vi "ReadSoundCard.vi"(3 "All Info":T1 {"Data Set"."Settings"."Time" format="%<%H:%M\n%d/%m/%y>T"; "task ID" format="%.0x"}) -> (0 "Data Set":T2[](array[typedef]) {"Settings"."Time" format="%<%H:%M\n%d/%m/%y>T"}, 1 "All Info":T1 {"Data Set"."Settings"."Time" format="%<%H:%M\n%d/%m/%y>T"; "task ID" format="%.0x"})   [LabVIEW 2014]
uses:
  <userlib>/CurtinCode/DataControl.ctl
  <userlib>/CurtinCode/SettingsControl.ctl
  <userlib>/CurtinCode/AllDataCtrl.ctl
  <vilib>/sound2/lvsound2.llb/Sound Input Task ID.ctl
  <vilib>/DAQmx/read.llb/DAQmx Read (Analog 1D Wfm NChan NSamp).vi
  <vilib>/sound2/lvsound2.llb/Sound Input Read (DBL).vi
panel:
  out "Waveform Graph":dbl[](graph)
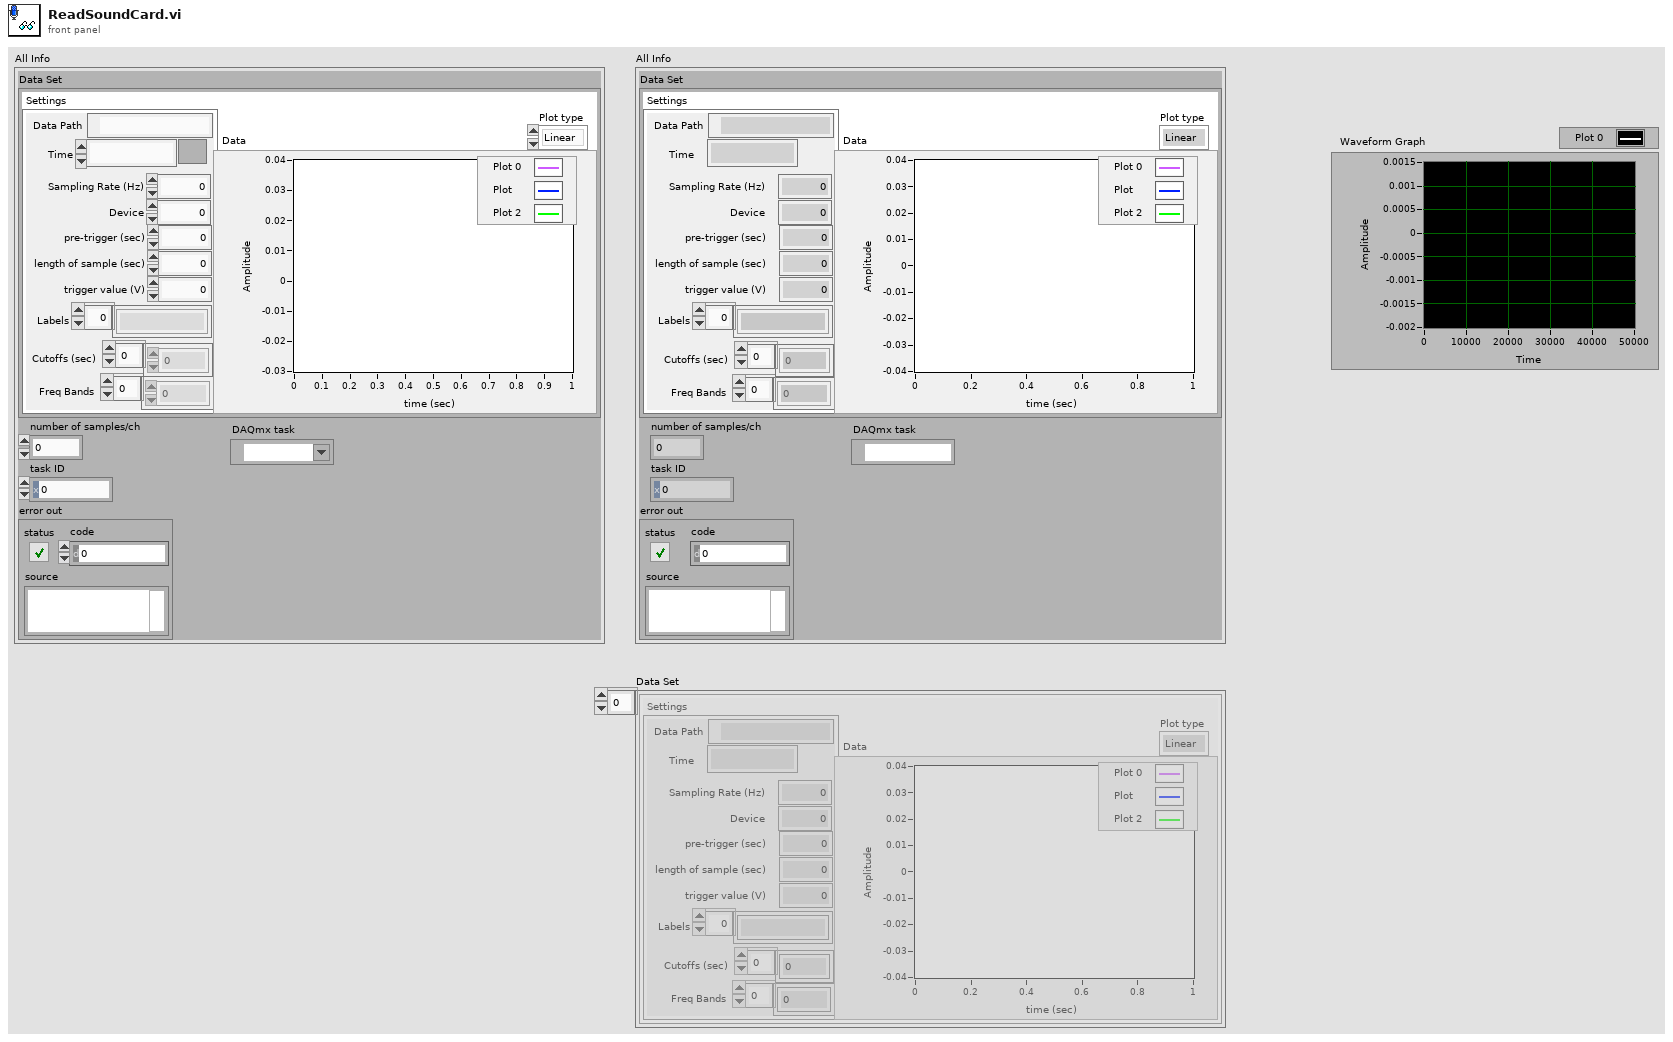
[diagram p1: front panel]
types:
  T1 = typedef "AllDataCtrl.ctl" = cluster{"Data Set":T2, "number of samples/ch":i32, "task ID":T4, "error out":errorcluster, "DAQmx task":refnum<k21>}
  T2 = typedef "DataControl.ctl" = cluster{"Settings":T3, "Data":cluster{i32, dbl, "data":dbl[]}[], "Plot type":enum16{"Linear", "log"}}
  T3 = typedef "SettingsControl.ctl" = cluster{"Data Path":path, "Time":timestamp, "Sampling Rate (Hz)":u16, "Device":u16, "pre-trigger (sec)":dbl, "length of sample (sec)":dbl, "trigger value (V)":dbl, "Labels":string[], "Cutoffs (sec)":dbl[], "Freq Bands":dbl[]}
  T4 = typedef "Sound Input Task ID.ctl" = u32
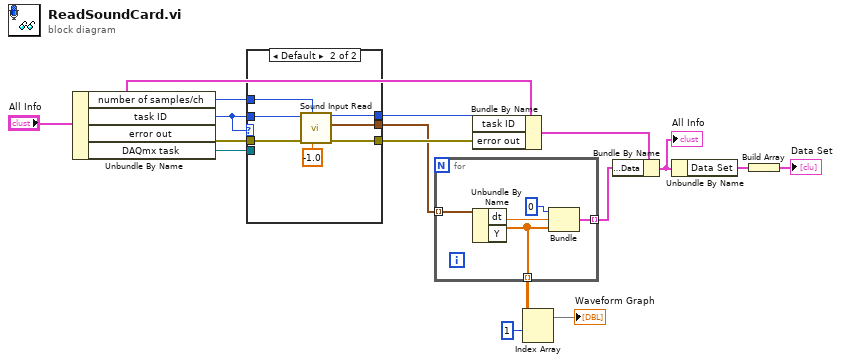
[diagram p0: block diagram]
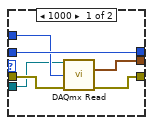
[diagram p2: hidden frame]
diagram:
  n1 = Unbundle By Name("All Info") -> ("number of samples/ch"=w4:i32, "task ID"=w6:T4, "error out"=w9:errorcluster, "DAQmx task"=w5:refnum<k21>)
  n2 = case shown="Default" w6 {
    tunnel: [w18 w29] -> w12
    tunnel: [w22 w28] -> w10
    tunnel: w9 -> [w19 w27]
    tunnel: w6 -> [w22 w26]
    tunnel: w4 -> [w20 w25]
    tunnel: [w21 w23] -> w7
    tunnel: w5 -> [w17 _]
    frame 1000 {
      n3 = call-poly <vilib>:"DAQmx Read.vi"("task/channels in"=w17, "number of samples per channel"=w20, "error in"=w19) -> ("data"=w21:waveform(dbl)[], "error out"=w18:errorcluster)  [unwired: 10 in, 1 out]
    }
    frame Default {
      n4 = call-poly <vilib>:"Sound Input Read.vi"("timeout (sec)"=-1.0, "number of samples/ch"=w25, "error in (no error)"=w27, "task ID"=w26) -> ("error out"=w29:errorcluster, "data"=w23:waveform(dbl)[], "task ID out"=w28:T4)  [unwired: 5 in]
    }
  }
  n5 = for {
    tunnel: w7 -> [w32] mode=indexing
    tunnel: [w33] -> w8 mode=indexing
    tunnel: [w30] -> w3 mode=indexing
    n6 = Unbundle By Name(w32) -> ("dt"=w31:dbl, "Y"=w30:dbl[])
    n7 = Bundle(0, "dt"=w31, "Y"=w30) -> (w33:cluster{i32, "dt":dbl, "Y":dbl[]})  [unwired: 1 in]
  }
  n8 = Bundle By Name(cluster="All Info", "task ID"=w10, "error out"=w12) -> (w13:T1)
  n9 = Index Array(array=w3, index (row)=1) -> (element=→"Waveform Graph":dbl[])  [unwired: 1 in]
  n10 = Bundle By Name(cluster=w13, "Data Set.Data"=w8) -> (w14:T1)
  "All Info" <- w14
  n11 = Unbundle By Name(w14) -> ("Data Set"=w15:T2)
  n12 = Build Array(w15) -> (→"Data Set":T2[])
